vi "EditOptions.vi"(8 "error in":errorcluster, 11 "node in":refnum<class "Targets.lvclass">) -> (0 "error out":errorcluster, 1 "edit options":T1, 2 "subnodes class":T2, 3 "node out":refnum<class "Targets.lvclass">)   [LabVIEW 2013, in "PL Framework Configuration Tool.lvlib" / "Targets.lvclass"]
doc: "Contains the options for the Menu that will be displayed when doing right click on an item.\nThe sub nodes class configures which nodes can be added to this nodes\nAnd the edit options determine which options are available for the node.\nThis configuration is stored in this VI in case some dynamic configuration is required for the menu options or sub nodes."
uses:
  Targets.lvclass
  <vilib>/NI/Configuration Framework/Node/SubNodeCluster.ctl
  <vilib>/NI/Configuration Framework/Node/NodeMenuOptions.ctl
  <vilib>/NI/Configuration Framework/Node/NISE_CEF_Node.lvclass/NISE_CEF_Node.ctl
  Engine Parent/Engine Parent Editor Node.lvclass
  Framework Configuration Classes/target configuration/PL_Target Configuration.lvclass/PL_Target Configuration.ctl
  Framework Configuration Classes/class cache/cache data.vi
  <vilib>/NI/Configuration Framework/Node/NISE_CEF_Node.lvclass
  Framework Configuration Classes/class cache/PL_class cache.lvlib
  Framework Configuration Classes/target configuration/PL_Target Configuration.lvclass
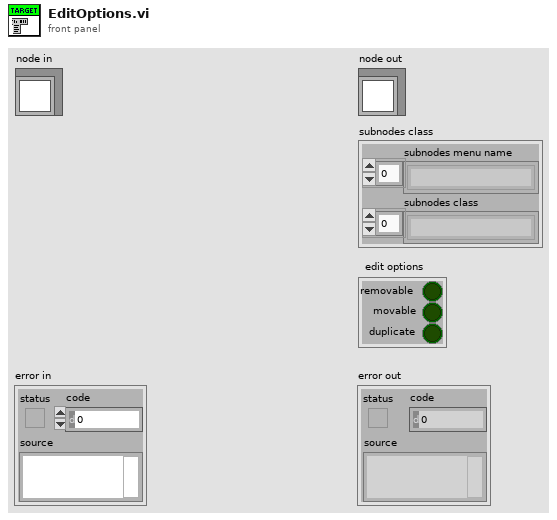
[diagram p1: front panel]
types:
  T1 = typedef "NISE_CEF_Node.lvclass/NodeMenuOptions.ctl" = cluster{"removable":bool, "movable":bool, "duplicate":bool}
  T2 = typedef "NISE_CEF_Node.lvclass/SubNodeCluster.ctl" = cluster{"subnodes menu name":string[], "subnodes class":string[]}
  T3 = typedef "NISE_CEF_Node.lvclass/NodeRef.ctl" = refnum<data-value>
  T4 = typedef "TBM configuration.lvclass/Target Types.ctl" = enum16{"Windows", "Mac", "Linux", "Linux RT ARM", "VxWorks", "Pharlap", "Other", "Linux RT x64"}
  T5 = typedef "PL_class cache.lvlib/cached class information.ctl" = cluster{"targets":T6[], "engines":T7[], "modules":T7[], "ignored class list":path[]}
  T6 = typedef "PL_class cache.lvlib/target class metadata.ctl" = cluster{"file name":string, "fully qualified name":string, "menu display name":string, "configuration class name":string}
  T7 = typedef "PL_class cache.lvlib/class metadata.ctl" = cluster{"file name":string, "fully qualified name":string, "menu display name":string, "configuration class":string, "instances allowed":i32, "supported targets":T4[]}
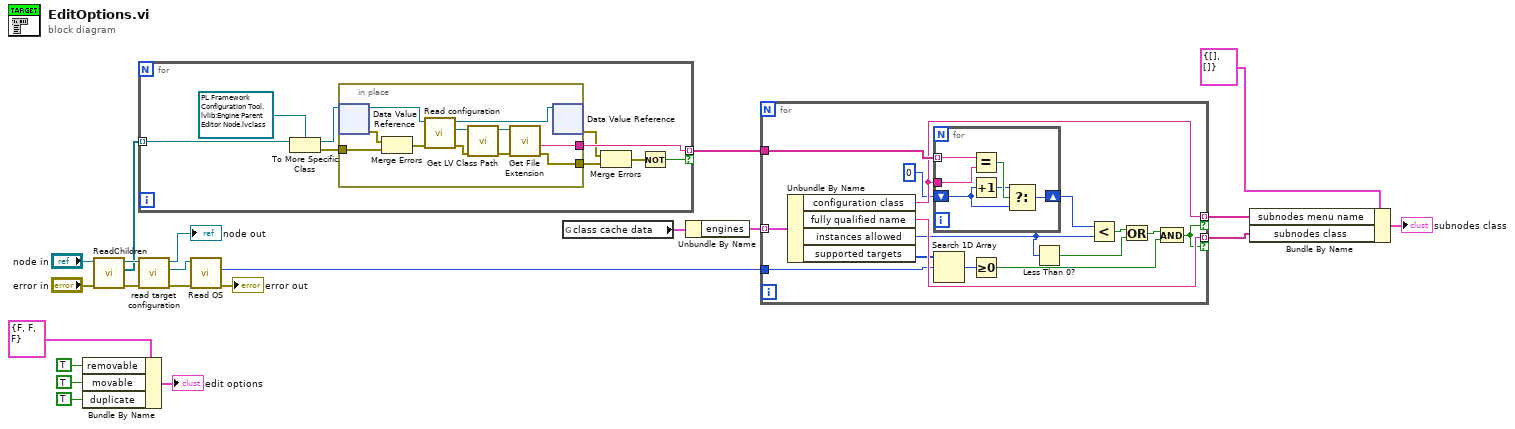
[diagram p0: block diagram]
diagram:
  n1 = Bundle By Name(cluster=T1 {"removable"=FALSE, "movable"=FALSE, "duplicate"=FALSE} ("edit options"), "removable"=TRUE ("Removable"), "movable"=TRUE ("Movable"), "duplicate"=TRUE ("Duplicate")) -> (→"edit options":T1)
  n2 = call <vilib>:"ReadChildren.vi"("error in"="error in", "node in"="node in") -> ("error out"=w8:errorcluster, "output array"=w3:T3[], "node out"=w9:refnum<class "Targets.lvclass">)  [unwired: 7 in]
  n3 = for {
    tunnel: w3 -> [w31] mode=indexing
    tunnel: [w27] -> w2 mode=indexing if=w23
    n4 = To More Specific Class(target class=refnum<data-value> refnum, reference=w31) -> (specific class reference=w29:refnum<data-value>, error out=w28:errorcluster)  [unwired: 1 in]
    n5 = in-place {
      in-place-border: w28 -> [w41]
      in-place-border: [w36] -> w27
      in-place-border: [w35] -> w25
      n6 = in-place-dvr #1(w29) -> (w34:refnum<class "Engine Parent Editor Node.lvclass">, w42:errorcluster)
      n7 = Merge Errors(w42, w41) -> (w33:errorcluster)
      n8 = call-dynamic "Read configuration.vi"("error in"=w33, "NISE_CEF_serializable node in"=w34) -> ("error out"=w39:errorcluster, "configuration"=w37:refnum<class "NISE_CEF_serializable configuration.lvclass">, "NISE_CEF_serializable node out"=w32:refnum<class "Engine Parent Editor Node.lvclass">)  [unwired: 7 in]
      n9 = call <vilib>:"Get LV Class Path.vi"("error in (no error)"=w39, "object"=w37) -> ("error out"=w38:errorcluster, "class path"=w40:path)  [unwired: 8 in]
      n10 = call <vilib>:"Get File Extension.vi"("error in (no error)"=w38, "file"=w40) -> ("error out"=w35:errorcluster, "filename without extension"=w36:string)  [unwired: 6 in, 2 out]
      n11 = in-place-dvr #1(w32) -> (w26:errorcluster)  [unwired: 1 out]
    }
    n12 = Merge Errors(w26, w25) -> (w24:errorcluster)
    n13 = Not(x=w24) -> (.not. x?=w23:bool)
  }
  n14 = call "read target configuration.vi"("error in"=w8, "Targets in"=w9) -> ("error out"=w7:errorcluster, "Target Configuration"=w4:refnum<class "PL_Target Configuration.lvclass">, "Targets out"=→"node out":refnum<class "Targets.lvclass">)  [unwired: 7 in]
  n15 = call "Read OS.vi"("error in"=w7, "PL_Target Configuration in"=w4) -> ("error out"=→"error out":errorcluster, "Target Types"=w1:T4)  [unwired: 7 in, 1 out]
  n16 = global read "cache data.vi" "class cache data"() -> (w13:T5)
  n17 = Unbundle By Name(w13) -> ("engines"=w12:T7[])
  n18 = for {
    tunnel: w12 -> [w57] mode=indexing
    tunnel: [w51] -> w17 mode=indexing if=w47
    tunnel: [w56] -> w16 mode=indexing if=w47
    tunnel: w2 -> [w52]
    tunnel: w1 -> [w54]
    n19 = Unbundle By Name(w57) -> ("configuration class"=w51:string, "fully qualified name"=w56:string, "instances allowed"=w44:i32, "supported targets"=w55:T4[])
    n20 = for {
      tunnel: w52 -> [w62] mode=indexing
      tunnel: w51 -> [w63]
      shift-right: [w58] -> w49
      shift-left: 0 -> [w59]
      n21 = Equal?(x=w62, y=w63) -> (x = y?=w61:bool)
      n22 = Increment(x=w59) -> (x+1=w60:i32)
      n23 = Select(t=w60, s=w61, f=w59) -> (s? t:f=w58:i32)
    }
    n24 = Search 1D Array(1D array=w55, element=w54) -> (index of element=w53:i32)  [unwired: 1 in]
    n25 = Greater Or Equal To 0?(x=w53) -> (x >= 0?=w48:bool)
    n26 = Less Than 0?(x=w44) -> (x < 0?=w43:bool)
    n27 = Less?(x=w49, y=w44) -> (x < y?=w46:bool)
    n28 = Or(x=w46, y=w43) -> (x .or. y?=w45:bool)
    n29 = And(x=w45, y=w48) -> (x .and. y?=w47:bool)
  }
  n30 = Bundle By Name(cluster=T2 {"subnodes menu name"=[], "subnodes class"=[]} ("subnodes class"), "subnodes menu name"=w17, "subnodes class"=w16) -> (→"subnodes class":T2)
